vi "Arrays{5th}.vi"() -> ()   [LabVIEW 2023]
panel:
  in  "index":i32
  out "element":dbl
  out "size(s)":i32
  out "Array 2":dbl[](array[slide]) scale=0.0..50.0
  in  "Array":dbl[](array[numeric])
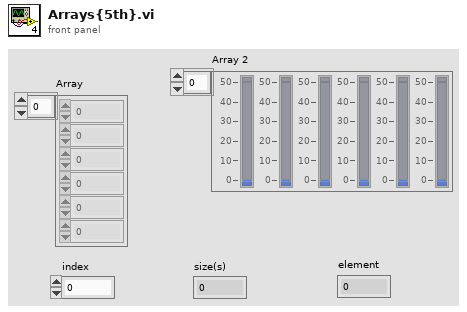
[diagram p1: front panel]
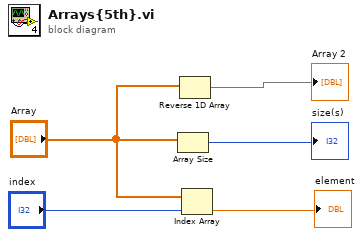
[diagram p0: block diagram]
diagram:
  n1 = Array Size(array="Array") -> (size(s)=→"size(s)":i32)
  n2 = Reverse 1D Array(array="Array") -> (reversed array=→"Array 2":dbl[])
  n3 = Index Array(array="Array", index="index") -> (element=→"element":dbl)
